vi "Compression with Wavelet (lossless).vi"() -> ()   [LabVIEW 2023]
doc: "This example shows the application of the integer wavelet transform (IWT) in lossless image compression.\n\nThe IWT converts integer signal samples or images into integer wavelet coefficients. You can compress these integer coefficients by entropy-based encoding without further quantization. As a result, you can reconstruct the original signal perfectly from a compressed set of IWT coefficients. \n\nThis example uses the WA Integer Wavelet Transform VI to compute the IWT coefficients of an image and reconstructs the image using the WA Inverse Integer Wavelet Transform VI. By comparing the difference between the original image and reconstructed image, this example shows that the IWT can achieve lossless image compression. In real-world compression applications, you can apply entropy-based encoding techniques such as the Huffman coding to the IWT coefficients of an image.\n\n<b>Instructions:</b>\n1) Run this VI.\n2) Select different images and observe the difference between the original and the reconstructed image."
uses:
  Images/_Images.ctl
  <vilib>/addons/Wavelet Analysis/discrete wavelet transform.llb/WA 2D Integer Wavelet Transform.vi
  <vilib>/addons/Wavelet Analysis/discrete wavelet transform.llb/WA Inverse 2D Integer Wavelet Transform.vi
  <vilib>/addons/_Advanced Signal Processing/NI_AdvSigProcWA.lvlib
panel:
  in  "Image":T1=enum."Part1"
  out "IWT Compressed, MiB":dbl format="%.2f"
  out "Equal":bool
  out "Raw image, MiB":dbl format="%.2f"
  out "Raw compressed, MiB":dbl format="%.2f"
  out "Reconstructed Image":T2(plugin-control)
  out "Original Image":T2(plugin-control)
  in  "Wavelet":u16(ring)=25 items=["Haar"=13, "bior2_2"=16, "bior4_4 (FBI)"=25]
  in  "Levels":i32=1
  # "Integer Wavelet Transform (IWT) - lossless image compression.\nAdvanced Signal Processing Toolkit is required"
  # "Compress Wavelet coefficients\ninstead of original image"
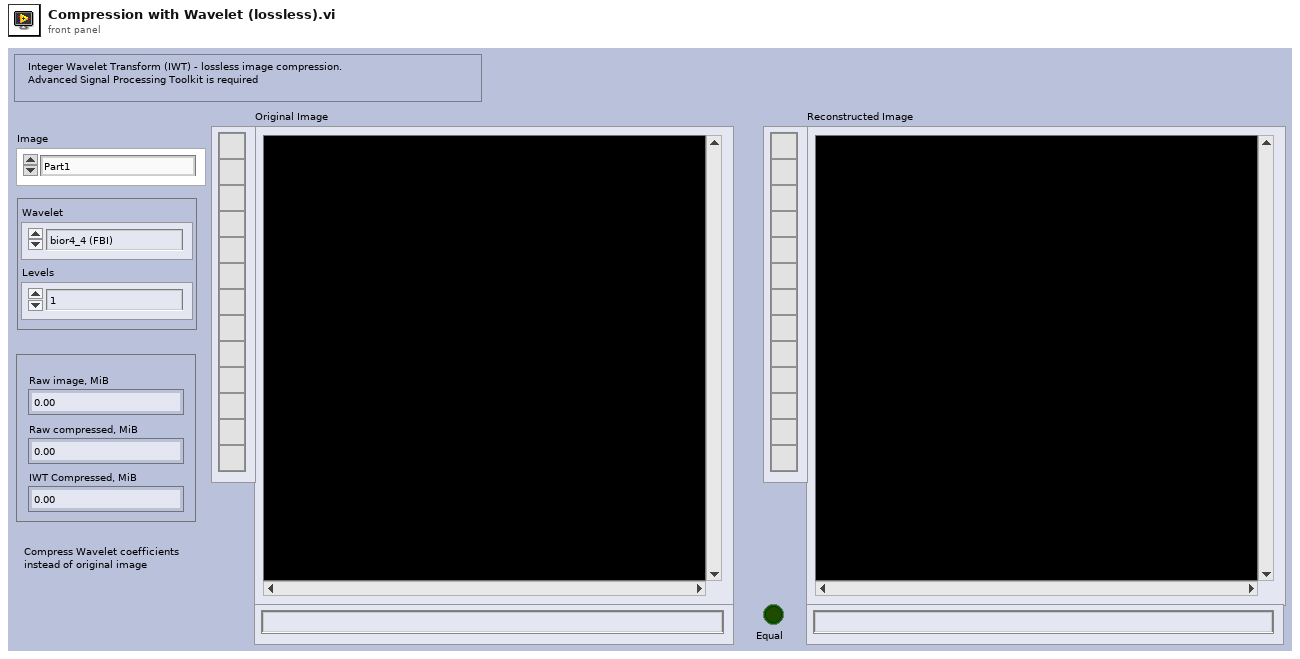
[diagram p1: front panel]
types:
  T1 = typedef "_Images.ctl" = enum16{"Ostern2023", "Balls2", "Battery1", "Battery2", "Connector1", "Subwoofer1", "Subwoofer2", "Subwoofer3", "Subwoofer4", "Hase1", "Lamp1", "Lamp2", "Mouse1", "PhotoLens1", "Po1", "PowerSupply1", "Router", "--- Step Wedges ---", "Stepwedge1", "Stepwedge2", "Stepwedge3", "--- Fusion ---", "Fusion160kV", "Fusion2-120kV", "Fusion2-320kV", "Fusion300kV", "FusionPart1-120kV", "FusionPart1-180kV", "--- PART 01 ---", "Part1", "Part2", "Part3", "Part4", "Part5", "Part6", "Part7", "Part8", "--- Different Integrations ---", "Step2737-02Int", "Step2737-04Int", "Step2737-08Int", "Step2737-16Int", "Step2737-32Int", "Step2737-64Int"}
  T2 = typedef "IMAQ Image.ctl" = refnum<image>
  T3 = typedef "Image Type" = u32
  T4 = cluster{"low_low":i32[][], "low_high":i32[][], "high_low":i32[][], "high_high":i32[][]}[]
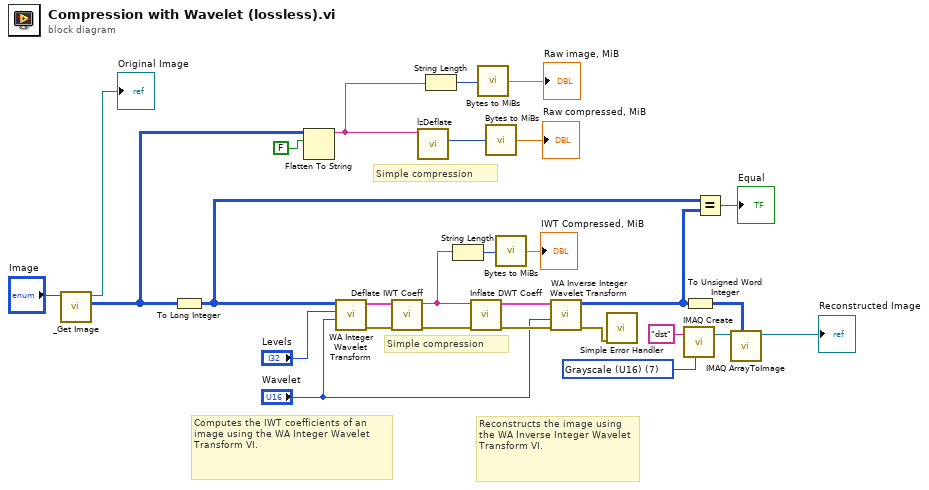
[diagram p0: block diagram]
diagram:
  w24 = T3 7 items=["Grayscale (U8)", "Grayscale (I16)", "Grayscale (SGL)", "Complex (CSG)", "RGB (U32)", "HSL (U32)", "RGB (U64)", "Grayscale (U16)"] ("Image Type")
  # "Simple compression"
  # "Simple compression"
  # "Reconstructs the image using the WA Inverse Integer Wavelet Transform VI."
  # "Computes the IWT coefficients of an image using the WA Integer Wavelet Transform VI."
  n1 = call "_Get Image.vi"("Image"="Image") -> ("Image Pixels (U16)"=w1:u16[][], "Image Out"=→"Original Image":T2)  [unwired: 7 in, 2 out]
  n2 = To Long Integer(number=w1) -> (32bit integer=w19:i32[][])
  n3 = Flatten To String(anything=w1, prepend array or string size? (T)=FALSE) -> (data string=w22:string)  [unwired: 2 in, 2 out]
  n4 = call-poly <vilib>:"WA Integer Wavelet Transform.vi"("wavelet"="Wavelet", "levels"="Levels", "signal"=w19) -> ("error out"=w13:errorcluster, "IWT coef"=w16:T4)  [unwired: 1 in, 6 out]
  n5 = call "Deflate IWT Coeff.vi"("error in (no error)"=w13, "IWT coef"=w16) -> ("error out"=w12:errorcluster, "data string"=w15:string)  [unwired: 7 in, 1 out]
  n6 = call "lzDeflate.vi"("input"=w22) -> ("length"=w7:i32)  [unwired: 4 in, 2 out]
  n7 = String Length(string=w22) -> (length=w9:i32)
  n8 = String Length(string=w15) -> (length=w5:i32)
  n9 = call "Inflate DWT Coeff.vi"("error in (no error)"=w12, "data string"=w15) -> ("error out"=w11:errorcluster, "Array"=w14:cluster{i32[][], i32[][], i32[][], i32[][]}[])  [unwired: 8 in]
  n10 = call "Bytes to MiBs.vi"("Numeric in"=w9) -> ("Numeric out"=→"Raw image, MiB":dbl)
  n11 = call "Bytes to MiBs.vi"("Numeric in"=w7) -> ("Numeric out"=→"Raw compressed, MiB":dbl)
  n12 = call "Bytes to MiBs.vi"("Numeric in"=w5) -> ("Numeric out"=→"IWT Compressed, MiB":dbl)
  n13 = call-poly <vilib>:"WA Inverse Integer Wavelet Transform.vi"("error in (no error)"=w11, "wavelet"="Wavelet", "IWT coef"=w14) -> ("error out"=w28:errorcluster, "signal"=w20:i32[][])  [unwired: 7 out]
  n14 = call <vilib>:"Simple Error Handler.vi"("error in (no error)"=w28) -> ()  [unwired: 1 in, 8 out]
  n15 = call "IMAQ Create"("Image Name"="dst", "Image Type"=w24) -> ("New Image"=w23:T2)  [unwired: 3 in, 1 out]
  n16 = To Unsigned Word Integer(number=w20) -> (unsigned 16bit integer=w17:u16[][])
  n17 = Equal?(x=w19, y=w20) -> (x = y?=→"Equal":bool)
  n18 = call "IMAQ ArrayToImage"("Image Pixels (U16)"=w17, "Image"=w23) -> ("Image Out"=→"Reconstructed Image":T2)  [unwired: 8 in, 1 out]
